vi "test_csm_interface.vi"() -> ()   [LabVIEW 2020]
uses:
  API/Create From VI Reference.vi
  Properties/Read User-Defined States.vi
  API/Destroy.vi
  CSM-Helper.lvclass
  <userlib>/_NEVSTOP/Communicable State Machine(CSM)/Communicable State Machine.lvlib
panel:
  out "resulting string":string
  out "error out":errorcluster
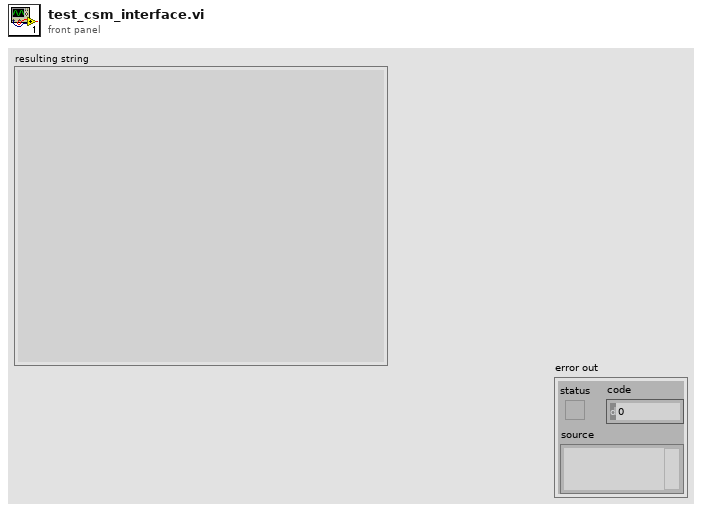
[diagram p1: front panel]
types:
  T1 = typedef "CSM-Helper.lvclass/Def-Argument Info.ctl" = cluster{"Type":string, "Name":string, "Variant":variant}
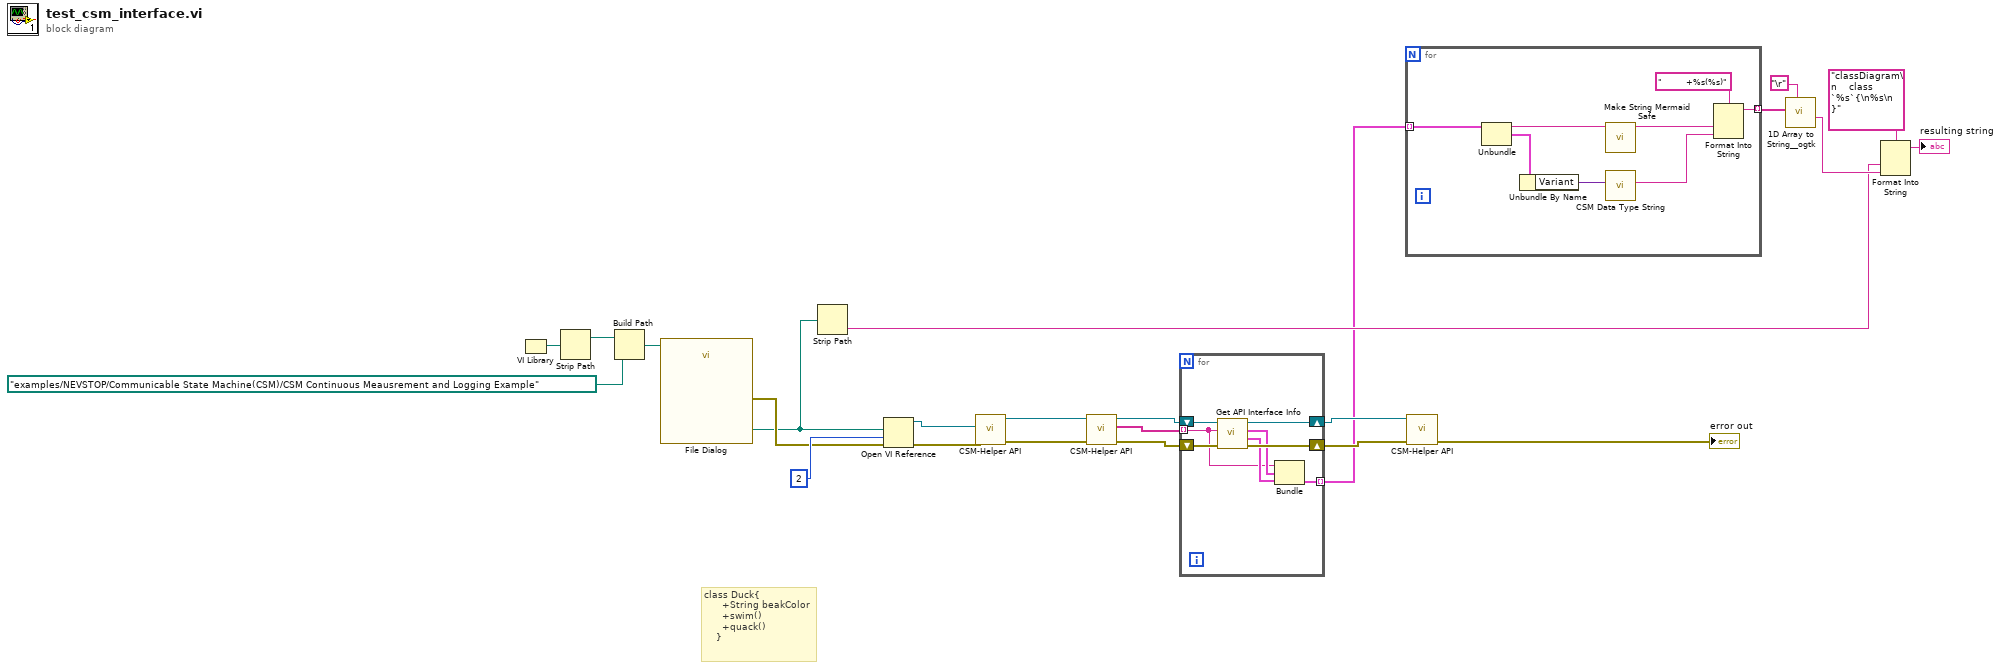
[diagram p0: block diagram]
diagram:
  # "class Duck{\n      +String beakColor\n      +swim()\n      +quack()\n    }"
  n1 = VI Library() -> (path=w24:path)
  n2 = Strip Path(path=w24) -> (stripped path=w23:path)  [unwired: 1 out]
  n3 = Build Path(base path=w23, name or relative path=path "examples/NEVSTOP/Communicable State Machine(CSM)/CSM Continuous Meausrement and Logging Example") -> (appended path=w21:path)
  n4 = call "File Dialog"("start path"=w21) -> ("selected path"=w11:path, "error out"=w16:errorcluster)  [unwired: 11 in, 2 out]
  n5 = Strip Path(path=w11) -> (name=w8:string)  [unwired: 1 out]
  n6 = Open VI Reference(vi path=w11, options=2, error in (no error)=w16) -> (vi reference=w17:refnum<vi>, error out=w18:errorcluster)  [unwired: 3 in]
  n7 = call-poly "CSM-Helper API.vi"("error in (no error)"=w18, "VI"=w17) -> ("error out"=w19:errorcluster, "CSM-Helper.lvclass"=w7:refnum<class "CSM-Helper.lvclass">)  [unwired: 8 in]
  n8 = call-poly "CSM-Helper API.vi"("error in (no error)"=w19, "CSM-Helper in"=w7) -> ("error out"=w6:errorcluster, "Array"=w2:string[], "CSM-Helper out"=w5:refnum<class "CSM-Helper.lvclass">)  [unwired: 7 in]
  n9 = for {
    shift-right: [w29] -> w3
    shift-left: w6 -> [w32]
    shift-right: [w30] -> w4
    shift-left: w5 -> [w31]
    tunnel: w2 -> [w25] mode=indexing
    tunnel: [w26] -> w1 mode=indexing
    n10 = call "Get API Interface Info.vi"("error in (no error)"=w32, "CASE"=w25, "CSM-Helper in"=w31) -> ("error out"=w29:errorcluster, "Response"=w28:T1, "Argument"=w27:T1, "CSM-Helper out"=w30:refnum<class "CSM-Helper.lvclass">)  [unwired: 5 in]
    n11 = Bundle(w25, "Argument"=w27, "Response"=w28) -> (w26:cluster{string, "Argument":T1, "Response":T1})  [unwired: 1 in]
  }
  n12 = for {
    tunnel: [w39] -> w14 mode=indexing
    tunnel: w1 -> [w37] mode=indexing
    n13 = Unbundle(w37) -> (w36:string, "Argument"=w35:T1)  [unwired: 1 out]
    n14 = Unbundle By Name(w35) -> ("Variant"=w34:variant)
    n15 = call "Make String Mermaid Safe.vi"("Source CSM"=w36) -> ("result string"=w38:string)  [unwired: 10 in]
    n16 = call <userlib>:"CSM Data Type String.vi"("Data"=w34) -> ("Data Type String"=w33:string)  [unwired: 10 in]
    n17 = Format Into String(format string="        +%s(%s)", w38, w33) -> (resulting string=w39:string)  [unwired: 2 in, 1 out]
  }
  n18 = call-poly "CSM-Helper API.vi"("error in (no error)"=w3, "CSM-Helper in"=w4) -> ("error out"=→"error out":errorcluster)  [unwired: 8 in, 1 out]
  n19 = call <userlib>:"1D Array to String__ogtk.vi"("delimiter (Tab)"="\r", "Array of Strings"=w14) -> ("delimited string"=w9:string)  [unwired: 9 in]
  n20 = Format Into String(format string="classDiagram\n    class `%s`{\n%s\n    }", w8, w9) -> (resulting string=→"resulting string":string)  [unwired: 2 in, 1 out]
